vi "Initialize_Parameters.vi"(6 "Files":T2, 7 "Timer parameters":refnum<vi>, 8 "Status/Errors in":refnum<vi>, 9 "Control parameters [] in":T25[](array[typedef]) {"Aux Byte Value" format="%02x"; "Max Real Value" format="%#_6e"; "Min Real Value" format="%#_6e"; "dReal/dByte" format="%#_6e"; "Byte Value" format="%02x"; "Identifier" format="%02x"}, 10 "Mode":T5={"Mode"=enum."Dialog", "Expert?"=FALSE, "Dialog?"=FALSE}, 11 "Data storage":T17 caption="Data Storage" {"Detector number" format="%#.0f"}) -> (0 "Status/Errors out":refnum<vi>, 1 "Control parameters [] out":T25[](array[typedef]) {"Aux Byte Value" format="%02x"; "Max Real Value" format="%#_6e"; "Min Real Value" format="%#_6e"; "dReal/dByte" format="%#_6e"; "Byte Value" format="%02x"; "Identifier" format="%02x"}, 2 "Main parameters":T4={"Mode"={"Mode"=enum."Dialog", "Expert?"=FALSE, "Dialog?"=FALSE}, "Stop loop"={"Settings changed?"=FALSE, "Stop?"=refnum}, "Send message"={"Send mode"=enum."Get parameters", "Set parameter list"=0, "Get parameter list"=0, "Reset device"=0, "Length set settings message"=0, "Reset buttons?"=FALSE, "Reset Master?"=enum."General"}, "Write settings"={"Options"=enum."File 1"}, "Settings state"={"MAS locked?"=refnum, "SLV locked?"=refnum}, "Button refs"={"Stop program"=refnum, "Save settings"=refnum, "DAQ mode"=refnum, "Reset settings"=refnum, "Apply settings"=refnum, "Reset MAS"=refnum, "Reset SLV"=refnum, "Local DBase?"=refnum, "Last value DBase"=FALSE, "Database"=refnum, "Calibration"=refnum, "Save settings 2"=refnum}, "Update screen"={"Detector number"=0, "Hardware"=enum."None"}, "Files"={"Path config file"=path "", "Path def. ini file"=path "", "Path ini file 1"=path "", "Path ini file 2"=path "", "Path RBF file"=path ""}, "DB connection"={"connection reference"=refnum, "Connected?"=refnum, "ODBC Name"=""}, "Status_id"=refnum, "Time difference"=refnum, "Satellites"=refnum, "Alignment parameters"=refnum, "Page Statistics 2"=refnum, "Database"=refnum, "Page Statistics"=refnum} {"Update screen"."Detector number" format="%#.0f"; "Send message"."Reset device" format="%x"; "Send message"."Get parameter list" format="%x"; "Send message"."Set parameter list" format="%x"}, 4 "Parameters":T20={"Mode"={"Mode"=enum."Dialog", "Expert?"=FALSE, "Dialog?"=FALSE}, "Stop loop"={"Settings changed?"=FALSE, "Stop?"=refnum}, "Send message"={"Send mode"=enum."Get parameters", "Set parameter list"=0, "Get parameter list"=0, "Reset device"=0, "Length set settings message"=0, "Reset buttons?"=FALSE, "Reset Master?"=enum."General"}, "Write settings"={"Options"=enum."File 1"}, "Read bytes"={"Max bytes read"=0, "Max bytes reached?"=FALSE}, "Settings state"={"MAS locked?"=refnum, "SLV locked?"=refnum}, "Button refs"={"Stop program"=refnum, "Save settings"=refnum, "DAQ mode"=refnum, "Reset settings"=refnum, "Apply settings"=refnum, "Reset MAS"=refnum, "Reset SLV"=refnum, "Local DBase?"=refnum, "Last value DBase"=FALSE, "Database"=refnum, "Calibration"=refnum, "Save settings 2"=refnum}, "Process messages"={"Process message mode"=enum."Error", "Slave data?"=FALSE, "Length get settings message"=0, "Delta time"=0.0, "Data_Filter"={"Filter_Data"=FALSE, "Use_Thresh"=FALSE, "Reduce data?"=FALSE}, "Time_difference_stack"=[], "Starting sec"=0, "Ending sec"=0, "Ending sec 2"=0, "MAS_Page_Thresh"=refnum, "SLV_Page_Thresh"=refnum, "Database"=refnum}, "Data storage"={"DB connection"={"connection reference"=refnum, "Connected?"=refnum, "ODBC Name"=""}, "Data storage condition"={"Database?"=FALSE}, "Detector number"=0, "# Messages to send"=0, "Database"=refnum, "Password"="", "Last error message"={"Last error message time stamp"={"Seconds"=0, "Minutes"=0, "Hours"=0, "Day"=0, "Month"=0, "Year"=0}, "Last error log"="", "Last error message"=""}, "Status_id"=refnum, "Hardware"=enum."None"}, "Update screen"={"Detector number"=0, "Hardware"=enum."None"}, "Alignment parameters"=refnum, "Timer parameters"=refnum, "Files"={"Path config file"=path "", "Path def. ini file"=path "", "Path ini file 1"=path "", "Path ini file 2"=path "", "Path RBF file"=path ""}, "Status_id"=refnum, "Time difference"=refnum, "Satellites"=refnum, "Calibration"={"GEN_Page_Calibrate"=refnum, "MAS_Page_Gain"=refnum, "MAS_Page_Offset"=refnum, "SLV_Page_Gain"=refnum, "SLV_Page_Offset"=refnum, "MAS_Page_Common"=refnum, "SLV_Page_Common"=refnum}, "Page Statistics 2"=refnum, "Page Statistics"=refnum} {"Update screen"."Detector number" format="%#.0f"; "Data storage"."Detector number" format="%#.0f"; "Read bytes"."Max bytes read" format="%#.0f"; "Send message"."Reset device" format="%x"; "Send message"."Get parameter list" format="%x"; "Send message"."Set parameter list" format="%x"})   [LabVIEW 2013]
uses:
  Controls/Control_Parameters.ctl
  Controls/Master.ctl
  Controls/Mode.ctl
  Controls/Parameters.ctl
  Controls/Stop_Loop.ctl
  Controls/Send_Message.ctl
  Controls/Send_Message_Mode.ctl
  Controls/Write_Settings.ctl
  Controls/Write_Settings_Options.ctl
  Controls/Read_Bytes.ctl
  Controls/Settings_State.ctl
  Controls/Button_Refs.ctl
  Controls/Process_Messages.ctl
  Controls/Process_Message_Mode.ctl
  Controls/Data_Storage.ctl
  Controls/DB_Connection.ctl
  database/Connection.llb/Conn ObjectReference.ctl
  Controls/Data_Storage_Condition.ctl
  Controls/GPS_Timestamp.ctl
  Controls/Update_Screen.ctl
  Controls/Files.ctl
  Controls/Page_Calibration.ctl
  Controls/Main_Parameters.ctl
  Controls/Calibration_Parameters.ctl
  Controls/Time_difference.ctl
  Controls/Get_Set_Statistics_Options2.ctl
panel:
  out "Status_id":u8
  out "Time difference":T1
  in  "Alignment parameters":T3 {"SLV Ch. 2"."Gain adjust neg." format="%02x"; "SLV Ch. 2"."Gain adjust pos." format="%02x"; "SLV Ch. 2"."Offset adjust neg." format="%02x"; "SLV Ch. 2"."Offset adjust pos." format="%02x"; "SLV Ch. 1"."Gain adjust neg." format="%02x"; "SLV Ch. 1"."Gain adjust pos." format="%02x"; "SLV Ch. 1"."Offset adjust neg." format="%02x"; "SLV Ch. 1"."Offset adjust pos." format="%02x"; "MAS Ch. 2"."Gain adjust neg." format="%02x"; "MAS Ch. 2"."Gain adjust pos." format="%02x"; "MAS Ch. 2"."Offset adjust neg." format="%02x"; "MAS Ch. 2"."Offset adjust pos." format="%02x"; "Full scale SLV" format="%02x"; "Comm. offset SLV" format="%02x"; "Coinc. time" format="%04x"; "Pre coinc. time" format="%04x"; "Post coinc. time" format="%04x"; "MAS Ch. 1"."Gain adjust neg." format="%02x"; "MAS Ch. 1"."Gain adjust pos." format="%02x"; "MAS Ch. 1"."Offset adjust neg." format="%02x"; "MAS Ch. 1"."Offset adjust pos." format="%02x"; "Full scale MAS" format="%02x"; "Comm. offset MAS" format="%02x"; "Trigger condition" format="%02x"}
  in  "Slave locked?":bool=TRUE
  in  "Master locked?":bool=TRUE
  in  "Stop?":bool
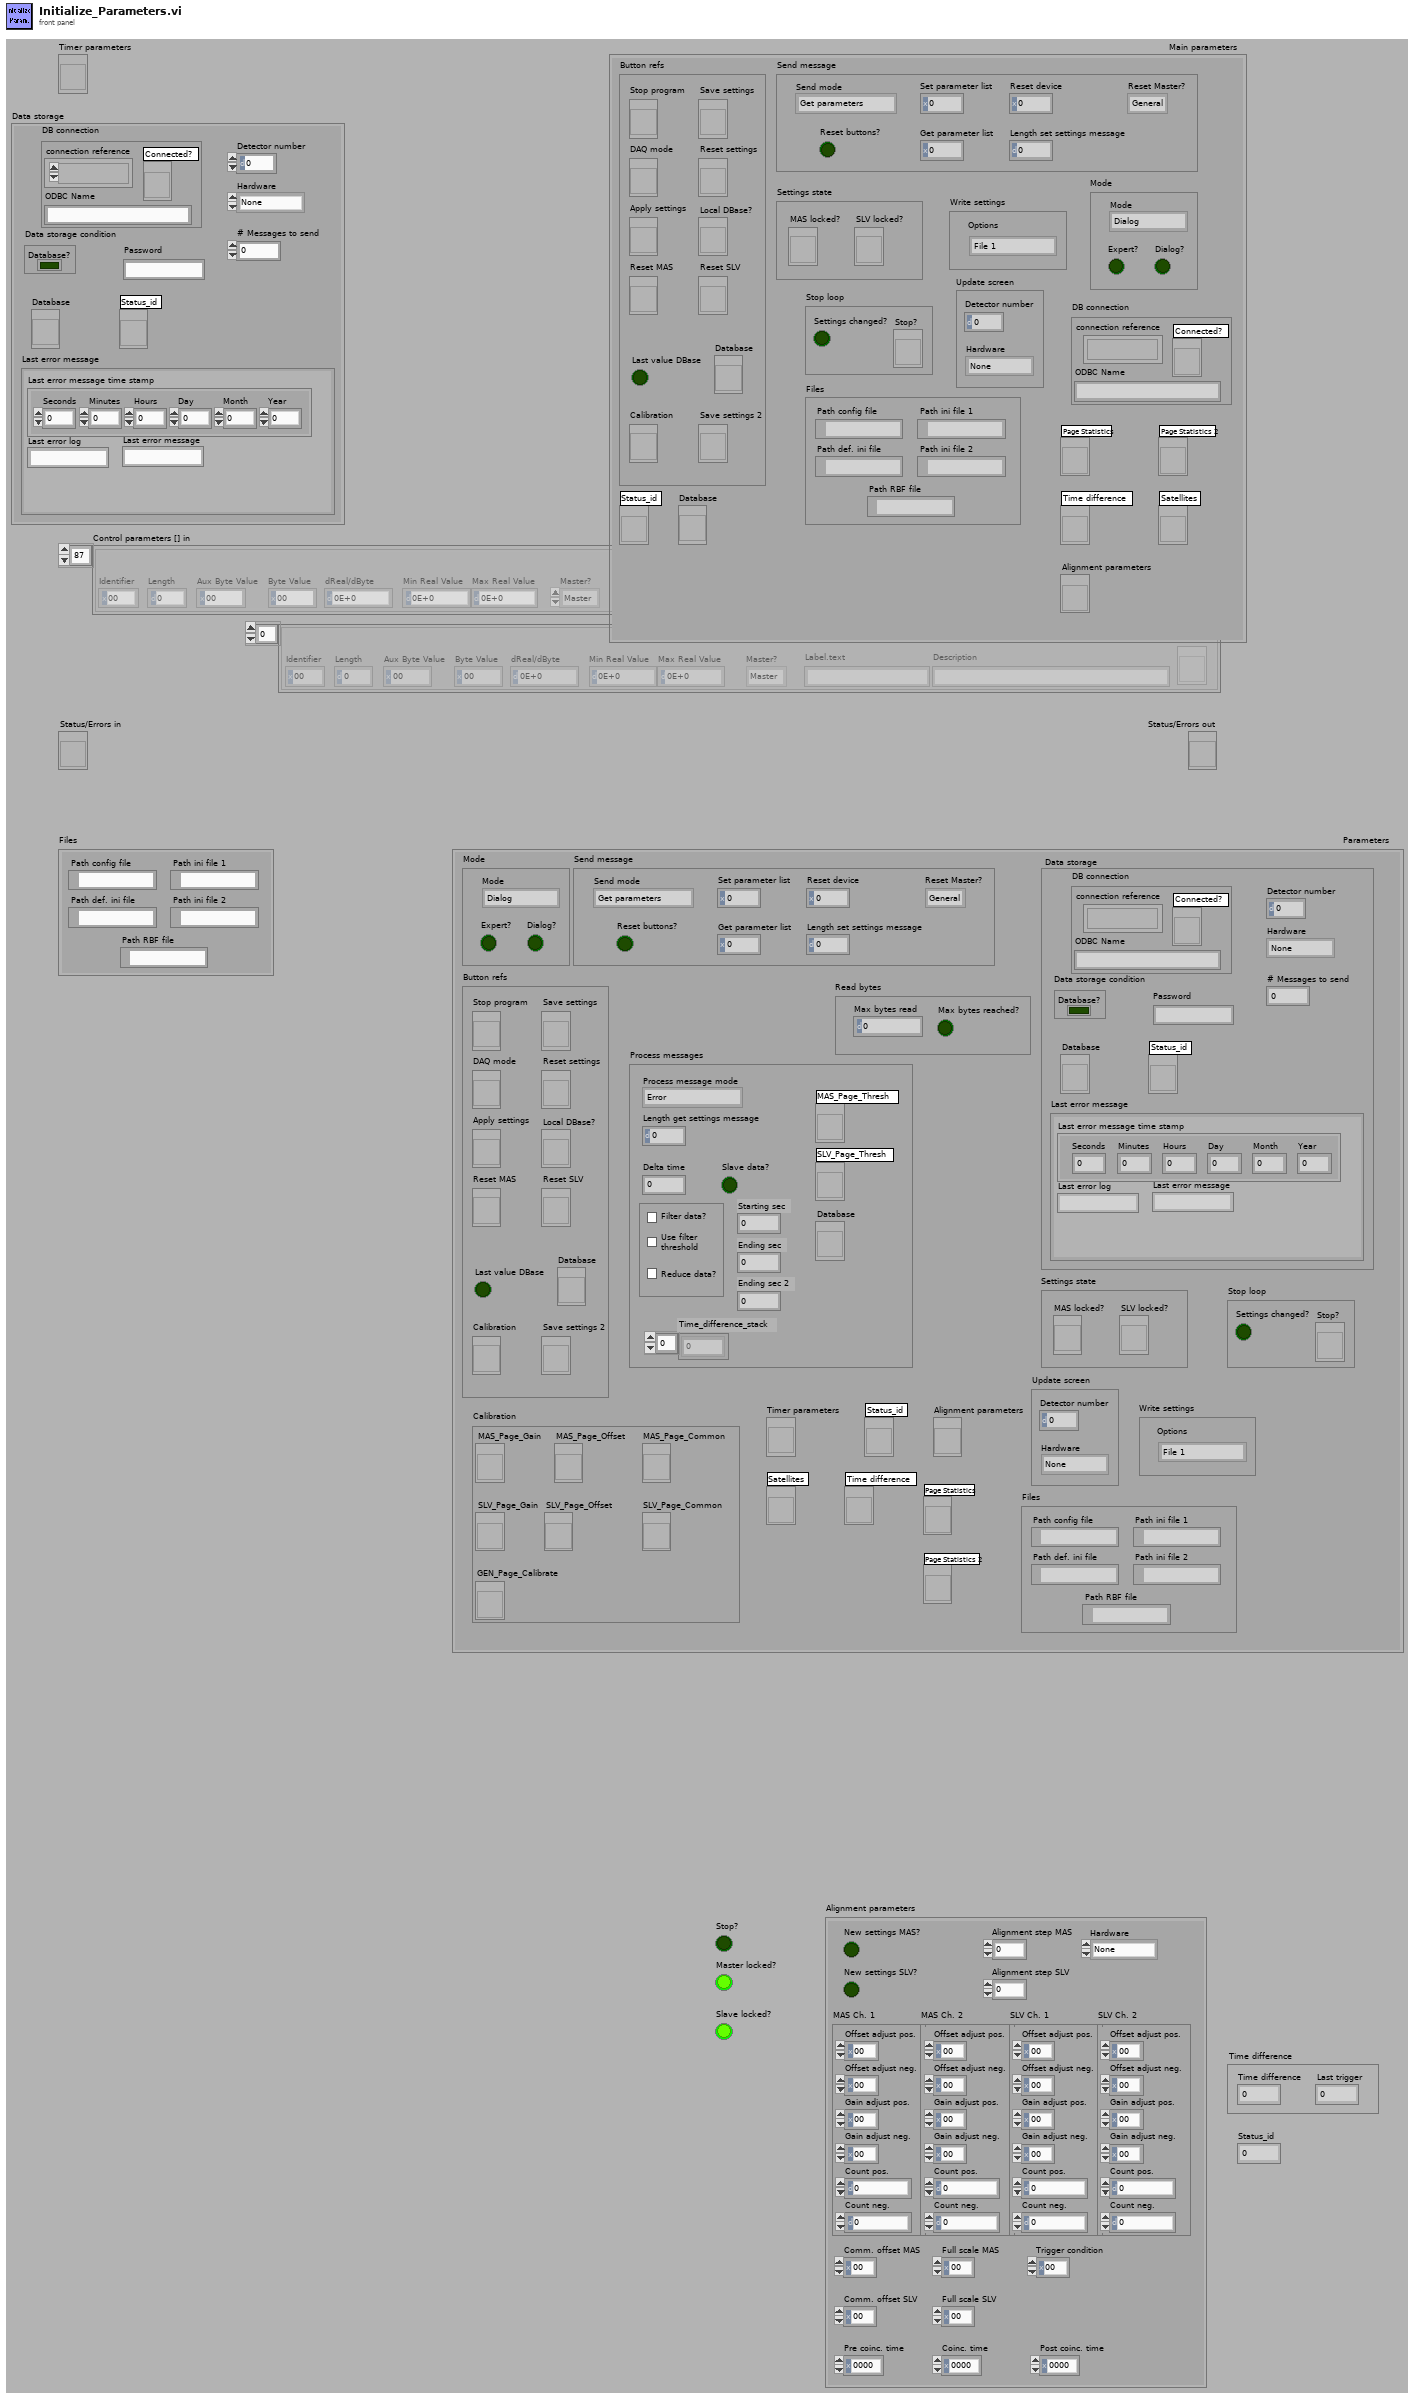
[diagram p1: front panel]
types:
  T1 = typedef "Time_difference.ctl" = cluster{"Last trigger":u64, "Time difference":u64}
  T2 = typedef "Files.ctl" = cluster{"Path config file":path, "Path def. ini file":path, "Path ini file 1":path, "Path ini file 2":path, "Path RBF file":path}
  T3 = typedef "Calibration_Parameters.ctl" = cluster{"New settings MAS?":bool, "New settings SLV?":bool, "Alignment step MAS":i32, "Alignment step SLV":i32, "MAS Ch. 1":cluster{"Offset adjust pos.":u8, "Offset adjust neg.":u8, "Gain adjust pos.":u8, "Gain adjust neg.":u8, "Count pos.":dbl, "Count neg.":dbl}, "MAS Ch. 2":cluster{"Offset adjust pos.":u8, "Offset adjust neg.":u8, "Gain adjust pos.":u8, "Gain adjust neg.":u8, "Count pos.":dbl, "Count neg.":dbl}, "SLV Ch. 1":cluster{"Offset adjust pos.":u8, "Offset adjust neg.":u8, "Gain adjust pos.":u8, "Gain adjust neg.":u8, "Count pos.":dbl, "Count neg.":dbl}, "SLV Ch. 2":cluster{"Offset adjust pos.":u8, "Offset adjust neg.":u8, "Gain adjust pos.":u8, "Gain adjust neg.":u8, "Count pos.":dbl, "Count neg.":dbl}, "Comm. offset MAS":u8, "Full scale MAS":u8, "Comm. offset SLV":u8, "Full scale SLV":u8, "Trigger condition":u8, "Pre coinc. time":u16, "Coinc. time":u16, "Post coinc. time":u16, "Hardware":enum8{"None", "HiSPARC I", "HiSPARC II", "HiSPARC III", "Unknown"}}
  T4 = typedef "Main_Parameters.ctl" = cluster{"Mode":T5, "Stop loop":T6, "Send message":T7, "Write settings":T10, "Settings state":T12, "Button refs":T13, "Update screen":T14, "Files":T2, "DB connection":T15, "Status_id":refnum<vi>, "Time difference":refnum<vi>, "Satellites":refnum<vi>, "Alignment parameters":refnum<vi>, "Page Statistics 2":refnum<vi>, "Database":refnum<vi>, "Page Statistics":refnum<vi>}
  T5 = typedef "Mode.ctl" = cluster{"Mode":enum8{"Stop", "Dialog", "Hisparc II", "Hisparc II DAQ", "Alignment"}, "Expert?":bool, "Dialog?":bool}
  T6 = typedef "Stop_Loop.ctl" = cluster{"Settings changed?":bool, "Stop?":refnum<vi>}
  T7 = typedef "Send_Message.ctl" = cluster{"Send mode":T8, "Set parameter list":u8, "Get parameter list":u8, "Reset device":u8, "Length set settings message":i32, "Reset buttons?":bool, "Reset Master?":T9}
  T8 = typedef "Send_Message_Mode.ctl" = enum16{"Get parameters", "Set parameters", "From front panel", "From parameters", "Reset device", "Alignment"}
  T9 = typedef "Master.ctl" = enum16{"Master", "Slave", "General"}
  T10 = typedef "Write_Settings.ctl" = cluster{"Options":T11}
  T11 = typedef "Write_Settings_Options.ctl" = enum16{"File 1", "File 2", "Alignment", "Reset"}
  T12 = typedef "Settings_State.ctl" = cluster{"MAS locked?":refnum<vi>, "SLV locked?":refnum<vi>}
  T13 = typedef "Button_Refs.ctl" = cluster{"Stop program":refnum<vi>, "Save settings":refnum<vi>, "DAQ mode":refnum<vi>, "Reset settings":refnum<vi>, "Apply settings":refnum<vi>, "Reset MAS":refnum<vi>, "Reset SLV":refnum<vi>, "Local DBase?":refnum<vi>, "Last value DBase":bool, "Database":refnum<vi>, "Calibration":refnum<vi>, "Save settings 2":refnum<vi>}
  T14 = typedef "Update_Screen.ctl" = cluster{"Detector number":u16, "Hardware":enum8{"None", "HiSPARC I", "HiSPARC II", "HiSPARC III", "Unknown"}}
  T15 = typedef "DB_Connection.ctl" = cluster{"connection reference":T16, "Connected?":refnum<vi>, "ODBC Name":string}
  T16 = typedef "Conn ObjectReference.ctl" = refnum<k1>
  T17 = typedef "Data_Storage.ctl" = cluster{"DB connection":T15, "Data storage condition":T18, "Detector number":u16, "# Messages to send":i32, "Database":refnum<vi>, "Password":string, "Last error message":cluster{"Last error message time stamp":T19, "Last error log":string, "Last error message":string}, "Status_id":refnum<vi>, "Hardware":enum8{"None", "HiSPARC I", "HiSPARC II", "HiSPARC III", "Unknown"}}
  T18 = typedef "Data_Storage_Condition.ctl" = cluster{"Database?":bool}
  T19 = typedef "GPS_Timestamp.ctl" = cluster{"Seconds":u8, "Minutes":u8, "Hours":u8, "Day":u8, "Month":u8, "Year":u16}
  T20 = typedef "Parameters.ctl" = cluster{"Mode":T5, "Stop loop":T6, "Send message":T7, "Write settings":T10, "Read bytes":T21, "Settings state":T12, "Button refs":T13, "Process messages":T22, "Data storage":T17, "Update screen":T14, "Alignment parameters":refnum<vi>, "Timer parameters":refnum<vi>, "Files":T2, "Status_id":refnum<vi>, "Time difference":refnum<vi>, "Satellites":refnum<vi>, "Calibration":T24, "Page Statistics 2":refnum<vi>, "Page Statistics":refnum<vi>}
  T21 = typedef "Read_Bytes.ctl" = cluster{"Max bytes read":u32, "Max bytes reached?":bool}
  T22 = typedef "Process_Messages.ctl" = cluster{"Process message mode":T23, "Slave data?":bool, "Length get settings message":i32, "Delta time":dbl, "Data_Filter":cluster{"Filter_Data":bool, "Use_Thresh":bool, "Reduce data?":bool}, "Time_difference_stack":u64[], "Starting sec":u64, "Ending sec":u64, "Ending sec 2":u64, "MAS_Page_Thresh":refnum<vi>, "SLV_Page_Thresh":refnum<vi>, "Database":refnum<vi>}
  T23 = typedef "Process_Message_Mode.ctl" = enum16{"Error", "Measurement data", "Comparator data", "One Second"}
  T24 = typedef "Page_Calibration.ctl" = cluster{"GEN_Page_Calibrate":refnum<vi>, "MAS_Page_Gain":refnum<vi>, "MAS_Page_Offset":refnum<vi>, "SLV_Page_Gain":refnum<vi>, "SLV_Page_Offset":refnum<vi>, "MAS_Page_Common":refnum<vi>, "SLV_Page_Common":refnum<vi>}
  T25 = typedef "Control_Parameters.ctl" = cluster{"Identifier":u8, "Length":u16, "Byte Value":u32, "dReal/dByte":dbl, "Min Real Value":dbl, "Max Real Value":dbl, "Master?":T9, "Label.text":string, "Description":string, "Refnum":refnum<vi>, "Aux Byte Value":u32}
  T26 = cluster{"Last trigger":u64, "Time difference":u64}
  T27 = typedef "Get_Set_Statistics_Options2.ctl" = enum16{"Get", "Set"}
  T28 = cluster{"Filter_Data":bool, "Use_Thresh":bool, "Reduce data?":bool}
  T29 = typedef "LVDateTimeRec.ctl" = cluster{"fractional second":dbl, "second":i32, "minute":i32, "hour":i32, "day of month":i32, "month":i32, "year":i32, "day of week":i32, "day of year":i32, "DST":i32}
  T30 = typedef "Page_Thresholds.ctl" = cluster{"Sing_Ch1_low":u32, "Sing_Ch1_high":u32, "Sing_Ch2_low":u32, "Sing_Ch2_high":u32, "Total_Ch1_low":u32, "Total_Ch1_high":u32, "Total_Ch2_low":u32, "Total_Ch2_high":u32, "Av_Ch1_low":dbl, "Av_Ch1_high":dbl, "Av_Ch2_low":dbl, "Av_Ch2_high":dbl}
  T31 = cluster{"Thresh_Count_MAS":T30, "Thresh_Count_SLV":T30, "Count":bool, "Time_to_count":u32, "Time":u32, "Time_to_count_ref":refnum<vi>, "Counting?":bool, "Baseline_MAS_Ch1":i16, "Baseline_MAS_Ch2":i16, "Baseline_SLV_Ch1":i16, "Baseline_SLV_Ch2":i16, "Basel_Err_MAS_Ch1":u32, "Basel_Err_MAS_Ch2":u32, "Basel_Err_SLV_Ch1":u32, "Basel_Err_SLV_Ch2":u32, "Peaks_Overshoot":dbl, "Height_Overshoot":dbl, "Integrals_Overshoot":dbl, "Last_event":dbl, "Total_Trigger":u32, "Av_Trigger":dbl, "Number of peaks":cluster{"t0":i32, "dt":i32, "Histogram":i32[][]}, "Pulse height":cluster{"t0":i32, "dt":i32, "Histogram":i32[][]}, "Integral":cluster{"t0":i32, "dt":i32, "Histogram":i32[][]}, "Number of peaks Entries":u64, "Number of peaks Overshoots":u64, "Pulse height  Entries":u64, "Pulse height Overshoots":u64, "Integral Entries":u64, "Integral Overshoots":u64, "Last trigger Stack":refnum<vi>}
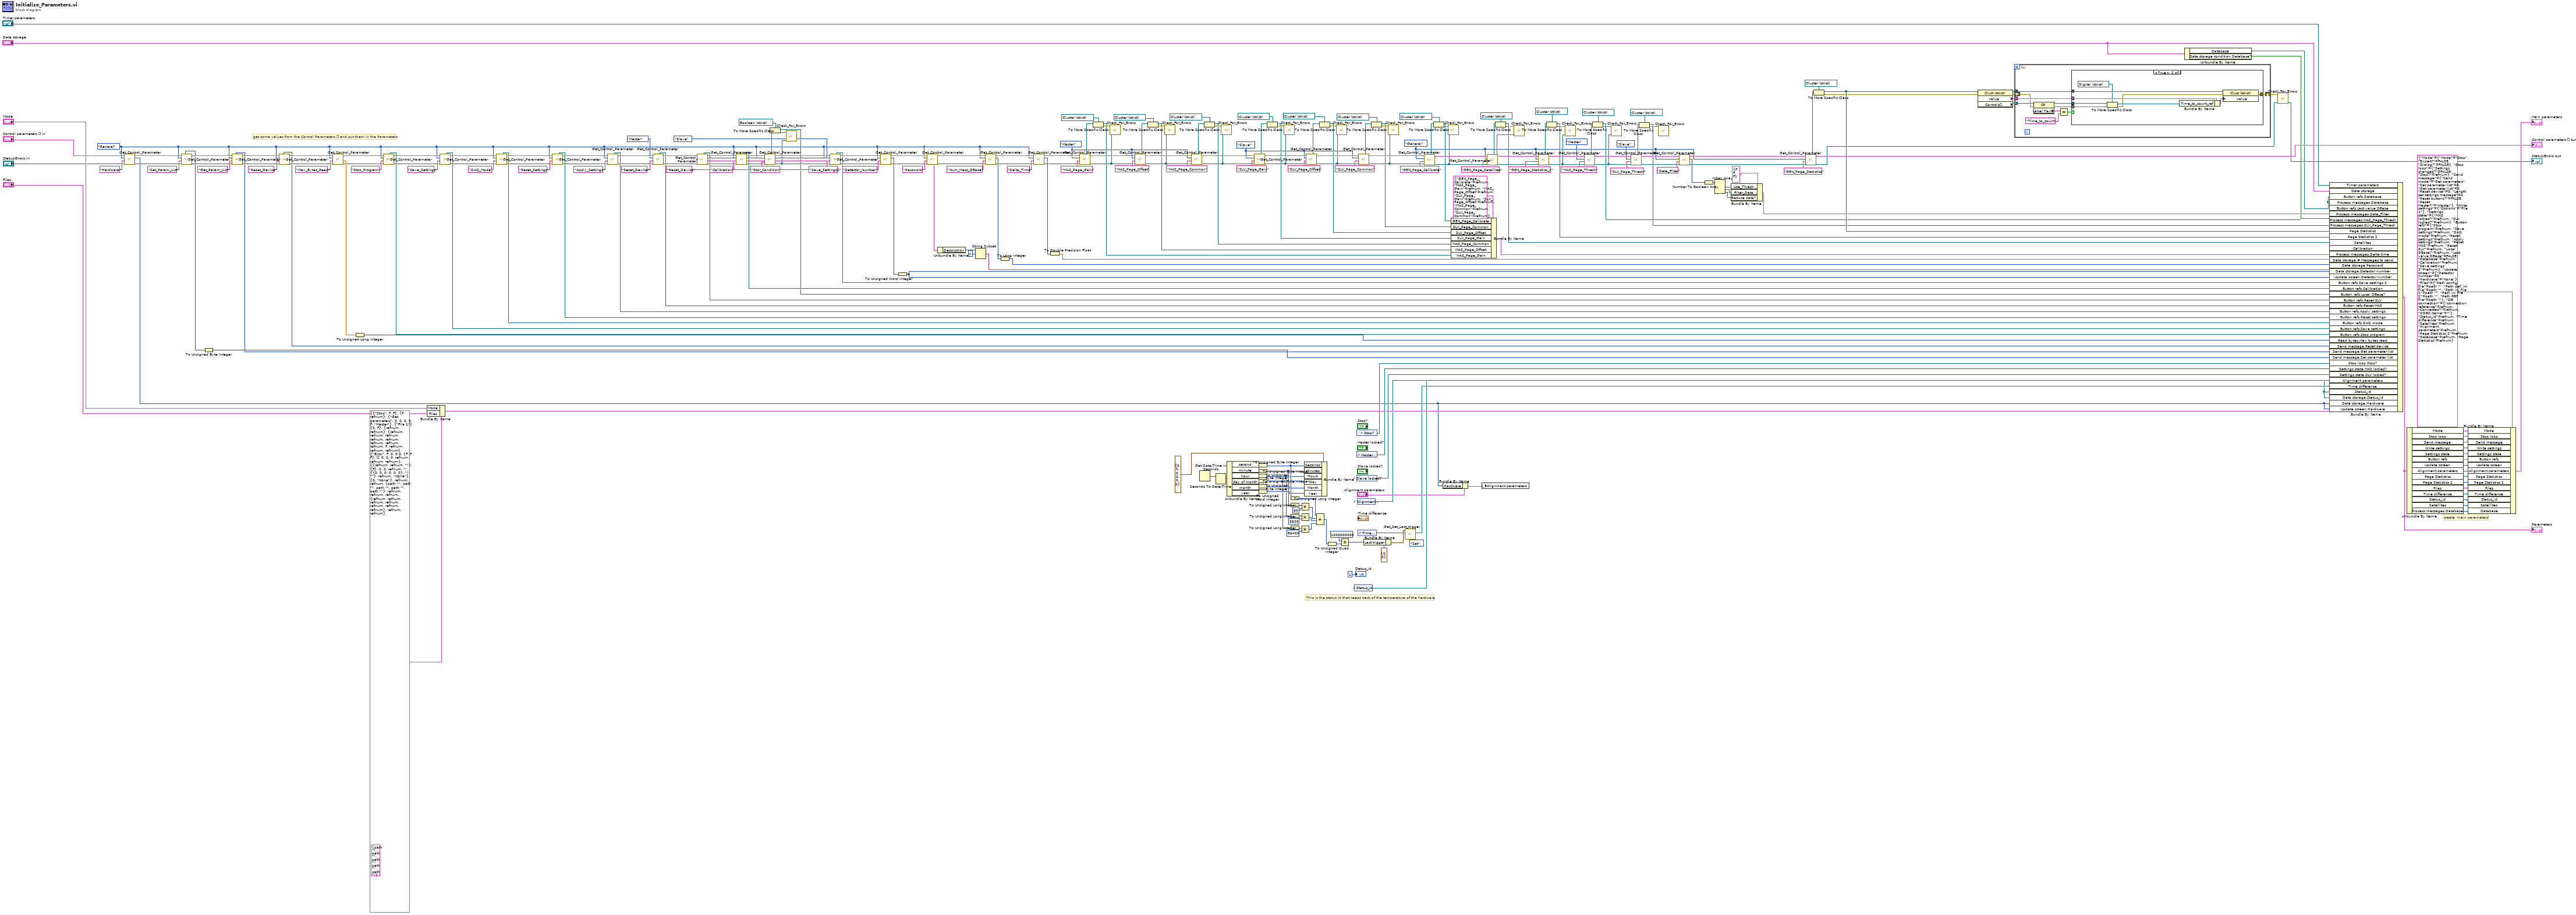
[diagram p0: block diagram]
diagram:
  w5 = Master."General" ("Master?")
  w77 = Master."General" ("Master?")
  w16 = Master."Slave" ("Master?")
  w30 = Master."Master" ("Master?")
  (unwired) T2 {"Path config file"=path "", "Path def. ini file"=path "", "Path ini file 1"=path "", "Path ini file 2"=path "", "Path RBF file"=path ""} ("Files")
  # "This is the status id that keeps track of the temperature of the hardware."
  # "create 'main parameters'"
  # "get some values from the Control Parameters [] and put them in the Parameters"
  n1 = call "Get_Control_Parameter.vi"("Status/Errors in"="Status/Errors in", "Label.text in"="Hardware", "Master?"=w5, "Control Parameters [] in"="Control parameters [] in") -> ("Status/Errors out"=w6:refnum<vi>, "Byte Value"=w2:u32, "Control Parameters [] out"=w4:T25[])  [unwired: 5 out]
  n2 = call "Get_Control_Parameter.vi"("Status/Errors in"=w6, "Label.text in"="Set_Param_List", "Master?"=w5, "Control Parameters [] in"=w4) -> ("Status/Errors out"=w264:refnum<vi>, "Control Parameters [] out"=w257:T25[], "Identifier"=w209:u8)  [unwired: 5 out]
  n3 = To Unsigned Byte Integer(number=w209) -> (unsigned 8bit integer=w262:u8)
  n4 = call "Get_Control_Parameter.vi"("Status/Errors in"=w264, "Label.text in"="Get_Param_List", "Master?"=w5, "Control Parameters [] in"=w257) -> ("Status/Errors out"=w263:refnum<vi>, "Control Parameters [] out"=w256:T25[], "Identifier"=w231:u8)  [unwired: 5 out]
  n5 = call "Get_Control_Parameter.vi"("Status/Errors in"=w263, "Label.text in"="Reset_Device", "Master?"=w5, "Control Parameters [] in"=w256) -> ("Status/Errors out"=w259:refnum<vi>, "Control Parameters [] out"=w255:T25[], "Identifier"=w232:u8)  [unwired: 5 out]
  n6 = call "Get_Control_Parameter.vi"("Status/Errors in"=w259, "Label.text in"="Max_Bytes_Read", "Master?"=w5, "Control Parameters [] in"=w255) -> ("Status/Errors out"=w248:refnum<vi>, "Real Value"=w260:dbl, "Control Parameters [] out"=w247:T25[])  [unwired: 5 out]
  n7 = To Unsigned Long Integer(number=w260) -> (unsigned 32bit integer=w258:u32)
  n8 = call "Get_Control_Parameter.vi"("Status/Errors in"=w248, "Label.text in"="Stop_Program", "Master?"=w5, "Control Parameters [] in"=w247) -> ("Status/Errors out"=w250:refnum<vi>, "Control Parameters [] out"=w249:T25[], "Refnum"=w235:refnum<vi>)  [unwired: 5 out]
  n9 = Bundle By Name(cluster=T20 {"Mode"={"Mode"=enum."Stop", "Expert?"=FALSE, "Dialog?"=FALSE}, "Stop loop"={"Settings changed?"=FALSE, "Stop?"=refnum}, "Send message"={"Send mode"=enum."Get parameters", "Set parameter list"=0, "Get parameter list"=0, "Reset device"=0, "Length set settings message"=0, "Reset buttons?"=FALSE, "Reset Master?"=enum."Master"}, "Write settings"={"Options"=enum."File 1"}, "Read bytes"={"Max bytes read"=0, "Max bytes reached?"=FALSE}, "Settings state"={"MAS locked?"=refnum, "SLV locked?"=refnum}, "Button refs"={"Stop program"=refnum, "Save settings"=refnum, "DAQ mode"=refnum, "Reset settings"=refnum, "Apply settings"=refnum, "Reset MAS"=refnum, "Reset SLV"=refnum, "Local DBase?"=refnum, "Last value DBase"=FALSE, "Database"=refnum, "Calibration"=refnum, "Save settings 2"=refnum}, "Process messages"={"Process message mode"=enum."Error", "Slave data?"=FALSE, "Length get settings message"=0, "Delta time"=0.0, "Data_Filter"={"Filter_Data"=FALSE, "Use_Thresh"=FALSE, "Reduce data?"=FALSE}, "Time_difference_stack"=[], "Starting sec"=0, "Ending sec"=0, "Ending sec 2"=0, "MAS_Page_Thresh"=refnum, "SLV_Page_Thresh"=refnum, "Database"=refnum}, "Data storage"={"DB connection"={"connection reference"=refnum, "Connected?"=refnum, "ODBC Name"=""}, "Data storage condition"={"Database?"=FALSE}, "Detector number"=0, "# Messages to send"=0, "Database"=refnum, "Password"="", "Last error message"={"Last error message time stamp"={"Seconds"=0, "Minutes"=0, "Hours"=0, "Day"=0, "Month"=0, "Year"=0}, "Last error log"="", "Last error message"=""}, "Status_id"=refnum, "Hardware"=enum."None"}, "Update screen"={"Detector number"=0, "Hardware"=enum."None"}, "Alignment parameters"=refnum, "Timer parameters"=refnum, "Files"={"Path config file"=path "", "Path def. ini file"=path "", "Path ini file 1"=path "", "Path ini file 2"=path "", "Path RBF file"=path ""}, "Status_id"=refnum, "Time difference"=refnum, "Satellites"=refnum, "Calibration"={"GEN_Page_Calibrate"=refnum, "MAS_Page_Gain"=refnum, "MAS_Page_Offset"=refnum, "SLV_Page_Gain"=refnum, "SLV_Page_Offset"=refnum, "MAS_Page_Common"=refnum, "SLV_Page_Common"=refnum}, "Page Statistics 2"=refnum, "Page Statistics"=refnum} ("Command parameters"), "Mode"="Mode", "Files"="Files") -> (w198:T20)
  n10 = call "Get_Control_Parameter.vi"("Status/Errors in"=w250, "Label.text in"="Save_Settings", "Master?"=w5, "Control Parameters [] in"=w249) -> ("Status/Errors out"=w241:refnum<vi>, "Control Parameters [] out"=w234:T25[], "Refnum"=w236:refnum<vi>)  [unwired: 5 out]
  n11 = call "Get_Control_Parameter.vi"("Status/Errors in"=w241, "Label.text in"="DAQ_Mode", "Master?"=w5, "Control Parameters [] in"=w234) -> ("Status/Errors out"=w244:refnum<vi>, "Control Parameters [] out"=w243:T25[], "Refnum"=w237:refnum<vi>)  [unwired: 5 out]
  n12 = call "Get_Control_Parameter.vi"("Status/Errors in"=w244, "Label.text in"="Reset_Settings", "Master?"=w5, "Control Parameters [] in"=w243) -> ("Status/Errors out"=w240:refnum<vi>, "Control Parameters [] out"=w233:T25[], "Refnum"=w238:refnum<vi>)  [unwired: 5 out]
  n13 = call "Get_Control_Parameter.vi"("Status/Errors in"=w240, "Label.text in"="Apply_Settings", "Master?"=w5, "Control Parameters [] in"=w233) -> ("Status/Errors out"=w204:refnum<vi>, "Control Parameters [] out"=w203:T25[], "Refnum"=w239:refnum<vi>)  [unwired: 5 out]
  n14 = call "Get_Control_Parameter.vi"("Status/Errors in"=w204, "Label.text in"="Reset_Device", "Master?"=Master."Master", "Control Parameters [] in"=w203) -> ("Status/Errors out"=w206:refnum<vi>, "Control Parameters [] out"=w205:T25[], "Refnum"=w199:refnum<vi>)  [unwired: 5 out]
  n15 = call "Get_Control_Parameter.vi"("Status/Errors in"=w206, "Label.text in"="Reset_Device", "Master?"=Master."Slave", "Control Parameters [] in"=w205) -> ("Status/Errors out"=w194:refnum<vi>, "Control Parameters [] out"=w195:T25[], "Refnum"=w200:refnum<vi>)  [unwired: 5 out]
  n16 = call "Get_Control_Parameter.vi"("Status/Errors in"=w194, "Label.text in"="Calibration", "Master?"=w5, "Control Parameters [] in"=w195) -> ("Status/Errors out"=w42:refnum<vi>, "Control Parameters [] out"=w41:T25[], "Refnum"=w193:refnum<vi>)  [unwired: 5 out]
  n17 = call "Get_Control_Parameter.vi"("Status/Errors in"=w42, "Label.text in"="Stor_Condition", "Master?"=w5, "Control Parameters [] in"=w41) -> ("Status/Errors out"=w43:refnum<vi>, "Control Parameters [] out"=w39:T25[], "Refnum"=w44:refnum<vi>)  [unwired: 5 out]
  n18 = To More Specific Class(target class=refnum<vi> refnum ("Button refs.Local DBase?"), reference=w44) -> (specific class reference=w40:refnum<vi>, error out=w45:errorcluster)  [unwired: 1 in]
  n19 = call "Check_For_Errors.vi"("Status/Errors in"=w43, "error in"=w45) -> ()  [unwired: 10 out]
  n20 = call "Get_Control_Parameter.vi"("Status/Errors in"=w43, "Label.text in"="Save_Settings2", "Master?"=w5, "Control Parameters [] in"=w39) -> ("Status/Errors out"=w162:refnum<vi>, "Control Parameters [] out"=w163:T25[], "Refnum"=w161:refnum<vi>)  [unwired: 5 out]
  n21 = call "Get_Control_Parameter.vi"("Status/Errors in"=w162, "Label.text in"="Detector_Number", "Master?"=w5, "Control Parameters [] in"=w163) -> ("Status/Errors out"=w179:refnum<vi>, "Byte Value"=w229:u32, "Control Parameters [] out"=w173:T25[])  [unwired: 5 out]
  n22 = To Unsigned Word Integer(number=w229) -> (unsigned 16bit integer=w171:u16)
  n23 = call "Get_Control_Parameter.vi"("Status/Errors in"=w179, "Label.text in"="Password", "Master?"=w5, "Control Parameters [] in"=w173) -> ("Status/Errors out"=w178:refnum<vi>, "Control Parameters [] out"=w172:T25[], "Control Parameter"=w177:T25)  [unwired: 5 out]
  n24 = Unbundle By Name(w177) -> ("Description"=w176:string)
  n25 = String Subset(string=w176, offset (0)=4) -> (substring=w174:string)  [unwired: 1 out]
  n26 = call "Get_Control_Parameter.vi"("Status/Errors in"=w178, "Label.text in"="Num_Mess_DBase", "Master?"=w5, "Control Parameters [] in"=w172) -> ("Status/Errors out"=w210:refnum<vi>, "Byte Value"=w228:u32, "Control Parameters [] out"=w212:T25[])  [unwired: 5 out]
  n27 = To Long Integer(number=w228) -> (32bit integer=w216:i32)
  n28 = call "Get_Control_Parameter.vi"("Status/Errors in"=w210, "Label.text in"="Delta_Time", "Master?"=w5, "Control Parameters [] in"=w212) -> ("Status/Errors out"=w84:refnum<vi>, "Byte Value"=w211:u32, "Control Parameters [] out"=w85:T25[])  [unwired: 5 out]
  n29 = To Double Precision Float(number=w211) -> (double precision float=w190:dbl)
  n30 = call "Get_Control_Parameter.vi"("Status/Errors in"=w84, "Label.text in"="MAS_Page_Gain", "Master?"=w30, "Control Parameters [] in"=w85) -> ("Status/Errors out"=w79:refnum<vi>, "Control Parameters [] out"=w78:T25[], "Refnum"=w88:refnum<vi>)  [unwired: 5 out]
  n31 = To More Specific Class(target class=refnum<vi> refnum ("MAS_Page_Gain"), reference=w88) -> (specific class reference=w10:refnum<vi>, error out=w54:errorcluster)  [unwired: 1 in]
  n32 = call "Check_For_Errors.vi"("Status/Errors in"=w79, "error in"=w54) -> ()  [unwired: 10 out]
  n33 = call "Get_Control_Parameter.vi"("Status/Errors in"=w79, "Label.text in"="MAS_Page_Offset", "Master?"=w30, "Control Parameters [] in"=w78) -> ("Status/Errors out"=w28:refnum<vi>, "Control Parameters [] out"=w22:T25[], "Refnum"=w86:refnum<vi>)  [unwired: 5 out]
  n34 = To More Specific Class(target class=refnum<vi> refnum ("MAS_Page_Offset"), reference=w86) -> (specific class reference=w11:refnum<vi>, error out=w55:errorcluster)  [unwired: 1 in]
  n35 = call "Check_For_Errors.vi"("Status/Errors in"=w28, "error in"=w55) -> ()  [unwired: 10 out]
  n36 = call "Get_Control_Parameter.vi"("Status/Errors in"=w28, "Label.text in"="MAS_Page_Common", "Master?"=w30, "Control Parameters [] in"=w22) -> ("Status/Errors out"=w27:refnum<vi>, "Control Parameters [] out"=w21:T25[], "Refnum"=w32:refnum<vi>)  [unwired: 5 out]
  n37 = Get Date/Time In Seconds() -> (seconds since 1Jan1904=w150:timestamp)
  n38 = To More Specific Class(target class=refnum<vi> refnum ("MAS_Page_Common"), reference=w32) -> (specific class reference=w12:refnum<vi>, error out=w33:errorcluster)  [unwired: 1 in]
  n39 = Seconds To Date/Time(time stamp (now)=w150) -> (date time rec=w149:T29)  [unwired: 1 out]
  n40 = call "Check_For_Errors.vi"("Status/Errors in"=w27, "error in"=w33) -> ()  [unwired: 10 out]
  n41 = Unbundle By Name(w149) -> ("second"=w147:i32, "minute"=w143:i32, "hour"=w144:i32, "day of month"=w145:i32, "month"=w146:i32, "year"=w141:i32)
  n42 = call "Get_Control_Parameter.vi"("Status/Errors in"=w27, "Label.text in"="SLV_Page_Gain", "Master?"=w16, "Control Parameters [] in"=w21) -> ("Status/Errors out"=w80:refnum<vi>, "Control Parameters [] out"=w81:T25[], "Refnum"=w83:refnum<vi>)  [unwired: 5 out]
  n43 = To Unsigned Byte Integer(number=w147) -> (unsigned 8bit integer=w126:u8)
  n44 = To Unsigned Byte Integer(number=w143) -> (unsigned 8bit integer=w125:u8)
  n45 = To Unsigned Byte Integer(number=w144) -> (unsigned 8bit integer=w124:u8)
  n46 = To Unsigned Byte Integer(number=w145) -> (unsigned 8bit integer=w123:u8)
  n47 = To Unsigned Byte Integer(number=w146) -> (unsigned 8bit integer=w140:u8)
  n48 = To Unsigned Word Integer(number=w141) -> (unsigned 16bit integer=w142:u16)
  n49 = To More Specific Class(target class=refnum<vi> refnum ("SLV_Page_Gain"), reference=w83) -> (specific class reference=w13:refnum<vi>, error out=w56:errorcluster)  [unwired: 1 in]
  n50 = call "Check_For_Errors.vi"("Status/Errors in"=w80, "error in"=w56) -> ()  [unwired: 10 out]
  n51 = To Unsigned Long Integer(number=w125) -> (unsigned 32bit integer=w134:u32)
  n52 = To Unsigned Long Integer(number=w124) -> (unsigned 32bit integer=w137:u32)
  n53 = To Unsigned Long Integer(number=w123) -> (unsigned 32bit integer=w135:u32)
  n54 = To Unsigned Long Integer(number=w126) -> (unsigned 32bit integer=w130:u32)
  n55 = Multiply(x=w134, y=u32 60) -> (x*y=w133:u32)
  n56 = Multiply(x=w137, y=u32 3600) -> (x*y=w132:u32)
  n57 = Multiply(x=w135, y=u32 86400) -> (x*y=w131:u32)
  n58 = Bundle By Name(cluster=T19 {"Seconds"=0, "Minutes"=0, "Hours"=0, "Day"=0, "Month"=0, "Year"=0} ("Last error message.Last error message time stamp"), "Seconds"=w126, "Minutes"=w125, "Hours"=w124, "Day"=w123, "Month"=w140, "Year"=w142) -> ()  [unwired: 1 out]
  n59 = call "Get_Control_Parameter.vi"("Status/Errors in"=w80, "Label.text in"="SLV_Page_Offset", "Master?"=w16, "Control Parameters [] in"=w81) -> ("Status/Errors out"=w18:refnum<vi>, "Control Parameters [] out"=w20:T25[], "Refnum"=w82:refnum<vi>)  [unwired: 5 out]
  n60 = Compound Arithmetic op=ADD(w130, w133, w132, w131) -> (w129:u32)
  n61 = To More Specific Class(target class=refnum<vi> refnum ("SLV_Page_Offset"), reference=w82) -> (specific class reference=w14:refnum<vi>, error out=w53:errorcluster)  [unwired: 1 in]
  n62 = To Unsigned Quad Integer(1:w129) -> (0:w128:u64)
  n63 = call "Check_For_Errors.vi"("Status/Errors in"=w18, "error in"=w53) -> ()  [unwired: 10 out]
  n64 = Multiply(x=u64 1000000000, y=w128) -> (x*y=w121:u64)
  n65 = control-ref of="Status_id"() -> (w111:refnum<vi>)
  n66 = control-ref of="Stop?"() -> (w226:refnum<vi>)
  n67 = control-ref of="Master locked?"() -> (w215:refnum<vi>)
  n68 = control-ref of="Slave locked?"() -> (w214:refnum<vi>)
  n69 = control-ref of="Alignment parameters"() -> (w192:refnum<vi>)
  n70 = control-ref of="Time difference"() -> (w114:refnum<vi>)
  n71 = call "Get_Control_Parameter.vi"("Status/Errors in"=w18, "Label.text in"="SLV_Page_Common", "Master?"=w16, "Control Parameters [] in"=w20) -> ("Status/Errors out"=w17:refnum<vi>, "Control Parameters [] out"=w19:T25[], "Refnum"=w25:refnum<vi>)  [unwired: 5 out]
  n72 = Bundle By Name(cluster=T26 {"Last trigger"=0, "Time difference"=0} ("Value out"), "Last trigger"=w121) -> (w118:T26)
  n73 = To More Specific Class(target class=refnum<vi> refnum ("MAS_Page_Common"), reference=w25) -> (specific class reference=w15:refnum<vi>, error out=w26:errorcluster)  [unwired: 1 in]
  n74 = call "Check_For_Errors.vi"("Status/Errors in"=w17, "error in"=w26) -> ()  [unwired: 10 out]
  n75 = call "Get_Set_Last_trigger.vi"("Get/Set"=Get_Set_Statistics_Options2."Set", "Time difference"=w114, "Value in"=w118) -> ("Time difference out"=w113:refnum<vi>)  [unwired: 1 in, 7 out]
  n76 = call "Get_Control_Parameter.vi"("Status/Errors in"=w17, "Label.text in"="GEN_Page_Calibrate", "Master?"=w77, "Control Parameters [] in"=w19) -> ("Status/Errors out"=w109:refnum<vi>, "Control Parameters [] out"=w107:T25[], "Refnum"=w188:refnum<vi>)  [unwired: 5 out]
  n77 = To More Specific Class(target class=refnum<vi> refnum ("GEN_Page_Calibrate"), reference=w188) -> (specific class reference=w73:refnum<vi>, error out=w52:errorcluster)  [unwired: 1 in]
  n78 = Bundle By Name(cluster="Alignment parameters", "Hardware"=w2) -> (w8:T3)
  n79 = call "Check_For_Errors.vi"("Status/Errors in"=w109, "error in"=w52) -> ()  [unwired: 10 out]
  n80 = Bundle By Name(cluster=T24 {"GEN_Page_Calibrate"=refnum, "MAS_Page_Gain"=refnum, "MAS_Page_Offset"=refnum, "SLV_Page_Gain"=refnum, "SLV_Page_Offset"=refnum, "MAS_Page_Common"=refnum, "SLV_Page_Common"=refnum} ("Calibration"), "GEN_Page_Calibrate"=w73, "SLV_Page_Common"=w15, "SLV_Page_Offset"=w14, "SLV_Page_Gain"=w13, "MAS_Page_Common"=w12, "MAS_Page_Offset"=w11, "MAS_Page_Gain"=w10) -> (w72:T24)
  n81 = local write "Alignment parameters"(w8) -> ()
  n82 = call "Get_Control_Parameter.vi"("Status/Errors in"=w109, "Label.text in"="GEN_Page_Satellites", "Master?"=w77, "Control Parameters [] in"=w107) -> ("Status/Errors out"=w106:refnum<vi>, "Control Parameters [] out"=w108:T25[], "Refnum"=w105:refnum<vi>)  [unwired: 5 out]
  n83 = To More Specific Class(target class=refnum<vi> refnum ("GEN_Page_Satellites"), reference=w105) -> (specific class reference=w89:refnum<vi>, error out=w51:errorcluster)  [unwired: 1 in]
  n84 = call "Check_For_Errors.vi"("Status/Errors in"=w106, "error in"=w51) -> ()  [unwired: 10 out]
  n85 = call "Get_Control_Parameter.vi"("Status/Errors in"=w106, "Label.text in"="GEN_Page_Statistics_2", "Master?"=w77, "Control Parameters [] in"=w108) -> ("Status/Errors out"=w97:refnum<vi>, "Control Parameters [] out"=w101:T25[], "Refnum"=w159:refnum<vi>)  [unwired: 5 out]
  n86 = To More Specific Class(target class=refnum<vi> refnum ("GEN_Page_Statistics_2"), reference=w159) -> (specific class reference=w154:refnum<vi>, error out=w50:errorcluster)  [unwired: 1 in]
  n87 = call "Check_For_Errors.vi"("Status/Errors in"=w97, "error in"=w50) -> ()  [unwired: 10 out]
  n88 = call "Get_Control_Parameter.vi"("Status/Errors in"=w97, "Label.text in"="MAS_Page_Thresh", "Master?"=Master."Master", "Control Parameters [] in"=w101) -> ("Status/Errors out"=w98:refnum<vi>, "Control Parameters [] out"=w75:T25[], "Refnum"=w102:refnum<vi>)  [unwired: 5 out]
  n89 = To More Specific Class(target class=refnum<vi> refnum ("MAS_Page_Thresh"), reference=w102) -> (specific class reference=w94:refnum<vi>, error out=w49:errorcluster)  [unwired: 1 in]
  n90 = call "Check_For_Errors.vi"("Status/Errors in"=w98, "error in"=w49) -> ()  [unwired: 10 out]
  n91 = call "Get_Control_Parameter.vi"("Status/Errors in"=w98, "Label.text in"="SLV_Page_Thresh", "Master?"=Master."Slave", "Control Parameters [] in"=w75) -> ("Status/Errors out"=w76:refnum<vi>, "Control Parameters [] out"=w74:T25[], "Refnum"=w99:refnum<vi>)  [unwired: 5 out]
  n92 = To More Specific Class(target class=refnum<vi> refnum ("SLV_Page_Thresh"), reference=w99) -> (specific class reference=w93:refnum<vi>, error out=w48:errorcluster)  [unwired: 1 in]
  n93 = call "Check_For_Errors.vi"("error in"=w48) -> ()  [unwired: 1 in, 10 out]
  n94 = call "Get_Control_Parameter.vi"("Status/Errors in"=w76, "Label.text in"="Data_Filter", "Master?"=w77, "Control Parameters [] in"=w74) -> ("Status/Errors out"=w61:refnum<vi>, "Byte Value"=w169:u32, "Control Parameters [] out"=w59:T25[])  [unwired: 5 out]
  n95 = Number To Boolean Array(number=w169) -> (Boolean array=w168:bool[])
  n96 = Index Array(array=w168) -> (element #1=w167:bool, element #2=w166:bool, element #3=w156:bool)  [unwired: 3 in]
  n97 = Bundle By Name(cluster=T28 {"Filter_Data"=FALSE, "Use_Thresh"=FALSE, "Reduce data?"=FALSE} ("Data_Filter"), "Use_Thresh"=w167, "Filter_Data"=w166, "Reduce data?"=w156) -> (w155:T28)
  n98 = call "Get_Control_Parameter.vi"("Status/Errors in"=w61, "Label.text in"="GEN_Page_Statistics", "Master?"=w77, "Control Parameters [] in"=w59) -> ("Status/Errors out"=w60:refnum<vi>, "Control Parameters [] out"=→"Control parameters [] out":T25[], "Refnum"=w186:refnum<vi>)  [unwired: 5 out]
  n99 = To More Specific Class(target class=refnum<vi> refnum ("GEN_Page_Statistics"), reference=w186) -> (specific class reference=w117:refnum<vi>, error out=w62:errorcluster)  [unwired: 1 in]
  n100 = property class="Clust (strict)"(reference=w117, error in=w62) -> (reference out=w183:refnum<vi>, error out=w182:errorcluster, "Value"=w184:T31, "Controls[]"=w185:refnum<vi>[])
  n101 = for {
    tunnel: w185 -> [w277] mode=indexing
    tunnel: w184 -> [w273]
    tunnel: w183 -> [w272]
    shift-right: [w268] -> w181
    shift-left: w182 -> [w270]
    n102 = property class="Ctl"(reference=w277, error in=w270) -> (reference out=w271:refnum<vi>, error out=w269:errorcluster, "Label.Text"=w276:string)
    n103 = Equal?(x=w276, y="Time_to_count") -> (x = y?=w274:bool)
    n104 = case shown="True" w274 {
      tunnel: w273 -> [_ w286]
      tunnel: w272 -> [_ w287]
      tunnel: w271 -> [_ w284]
      tunnel: w269 -> [w278 w283]
      tunnel: [w278 w280] -> w268
      frame False {
      }
      frame True {
        n105 = To More Specific Class(target class=refnum<vi> refnum ("Time_to_count_ref"), reference=w284, error in=w283) -> (specific class reference=w282:refnum<vi>, error out=w281:errorcluster)
        n106 = Bundle By Name(cluster=w286, "Time_to_count_ref"=w282) -> (w285:T31)
        n107 = property class="Clust (strict)"(reference=w287, error in=w281, "Value"=w285) -> (error out=w280:errorcluster)  [unwired: 1 out]
      }
    }
  }
  n108 = Unbundle By Name("Data storage") -> ("Database"=w36:refnum<vi>, "Data storage condition.Database?"=w151:bool)
  n109 = call "Check_For_Errors.vi"("Status/Errors in"=w60, "error in"=w181) -> ("Status/Errors out"=→"Status/Errors out":refnum<vi>)  [unwired: 9 out]
  n110 = Bundle By Name(cluster=w198, "Timer parameters"="Timer parameters", "Data storage"="Data storage", "Button refs.Database"=w36, "Process messages.Database"=w36, "Button refs.Last value DBase"=w151, "Process messages.Data_Filter"=w155, "Process messages.MAS_Page_Thresh"=w94, "Process messages.SLV_Page_Thresh"=w93, "Page Statistics"=w117, "Page Statistics 2"=w154, "Satellites"=w89, "Calibration"=w72, "Process messages.Delta time"=w190, "Data storage.# Messages to send"=w216, "Data storage.Password"=w174, "Data storage.Detector number"=w171, "Update screen.Detector number"=w171, "Button refs.Save settings 2"=w161, "Button refs.Calibration"=w193, "Button refs.Local DBase?"=w40, "Button refs.Reset SLV"=w200, "Button refs.Reset MAS"=w199, "Button refs.Apply settings"=w239, "Button refs.Reset settings"=w238, "Button refs.DAQ mode"=w237, "Button refs.Save settings"=w236, "Button refs.Stop program"=w235, "Read bytes.Max bytes read"=w258, "Send message.Reset device"=w232, "Send message.Get parameter list"=w231, "Send message.Set parameter list"=w262, "Stop loop.Stop?"=w226, "Settings state.MAS locked?"=w215, "Settings state.SLV locked?"=w214, "Alignment parameters"=w192, "Time difference"=w113, "Status_id"=w111, "Data storage.Status_id"=w111, "Data storage.Hardware"=w2, "Update screen.Hardware"=w2) -> (w218:T20)
  "Parameters" <- w218
  n111 = Unbundle By Name(w218) -> ("Mode"=w224:T5, "Stop loop"=w223:T6, "Send message"=w222:T7, "Write settings"=w221:T10, "Settings state"=w220:T12, "Button refs"=w219:T13, "Update screen"=w197:T14, "Alignment parameters"=w191:refnum<vi>, "Page Statistics"=w34:refnum<vi>, "Page Statistics 2"=w112:refnum<vi>, "Files"=w158:T2, "Time difference"=w122:refnum<vi>, "Status_id"=w116:refnum<vi>, "Satellites"=w104:refnum<vi>, "Process messages.Database"=w37:refnum<vi>)
  n112 = Bundle By Name(cluster=T4 {"Mode"={"Mode"=enum."Stop", "Expert?"=FALSE, "Dialog?"=FALSE}, "Stop loop"={"Settings changed?"=FALSE, "Stop?"=refnum}, "Send message"={"Send mode"=enum."Get parameters", "Set parameter list"=0, "Get parameter list"=0, "Reset device"=0, "Length set settings message"=0, "Reset buttons?"=FALSE, "Reset Master?"=enum."Master"}, "Write settings"={"Options"=enum."File 1"}, "Settings state"={"MAS locked?"=refnum, "SLV locked?"=refnum}, "Button refs"={"Stop program"=refnum, "Save settings"=refnum, "DAQ mode"=refnum, "Reset settings"=refnum, "Apply settings"=refnum, "Reset MAS"=refnum, "Reset SLV"=refnum, "Local DBase?"=refnum, "Last value DBase"=FALSE, "Database"=refnum, "Calibration"=refnum, "Save settings 2"=refnum}, "Update screen"={"Detector number"=0, "Hardware"=enum."None"}, "Files"={"Path config file"=path "", "Path def. ini file"=path "", "Path ini file 1"=path "", "Path ini file 2"=path "", "Path RBF file"=path ""}, "DB connection"={"connection reference"=refnum, "Connected?"=refnum, "ODBC Name"=""}, "Status_id"=refnum, "Time difference"=refnum, "Satellites"=refnum, "Alignment parameters"=refnum, "Page Statistics 2"=refnum, "Database"=refnum, "Page Statistics"=refnum} ("Main parameters"), "Mode"=w224, "Stop loop"=w223, "Send message"=w222, "Write settings"=w221, "Settings state"=w220, "Button refs"=w219, "Update screen"=w197, "Alignment parameters"=w191, "Page Statistics"=w34, "Page Statistics 2"=w112, "Files"=w158, "Time difference"=w122, "Status_id"=w116, "Satellites"=w104, "Database"=w37) -> (→"Main parameters":T4)
  "Status_id" <- u8 1 ("Status_id")
